vi "Set Laser Power.vi"(6 "Mode":enum16{"Normal", "Ignore", "Reset"}(ring), 7 "Correlation ID":u32, 8 "error in (no error)":errorcluster, 9 "Power":dbl, 10 "laser index":u16, 11 "Application in":refnum<class "Application.lvclass">) -> (0 "error out":errorcluster, 3 "Application out":refnum<class "Application.lvclass">)   [LabVIEW 2023, in "Application.lvlib" / "Application.lvclass"]
uses:
  Application.lvclass
  Application.lvclass/Application.ctl
  Hardware/Device Messages/Save CorrID Msg/Save CorrID Msg.lvclass/Save CorrID Msg.ctl
  <vilib>/ActorFramework/Message Enqueuer/Message Enqueuer.lvclass/Message Enqueuer.ctl
  Hardware/Laser Messages/Set Power Msg/Set Power Msg.lvclass/Set Power Msg.ctl
  <vilib>/ActorFramework/Message Enqueuer/Enqueue.vi
  Hardware/Device Messages/Save CorrID Msg/Save CorrID Msg.lvclass
  Hardware/Laser Messages/Set Power Msg/Set Power Msg.lvclass
  <vilib>/ActorFramework/Message Priority Queue/Priority Enqueue.vi
  Application.lvlib
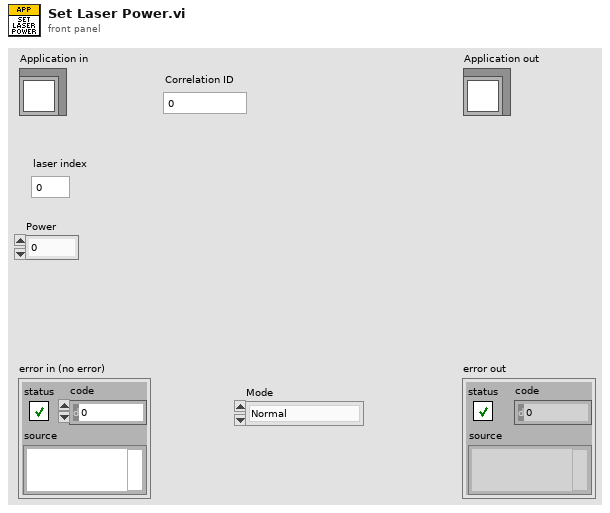
[diagram p1: front panel]
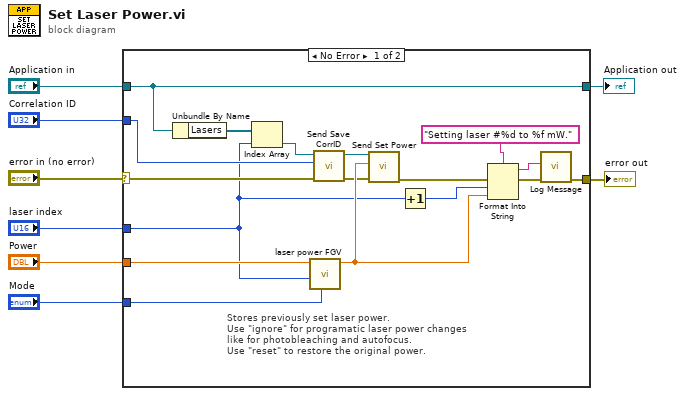
[diagram p0: block diagram]
diagram:
  n1 = case shown="No Error" "error in (no error)" {
    selector: "error in (no error)" -> [w15 w27]
    tunnel: [w22 w27] -> w7
    tunnel: [w12 w26] -> w5
    tunnel: "Application in" -> [w12 w26]
    tunnel: "Power" -> [w25 _]
    tunnel: "laser index" -> [w9 _]
    tunnel: "Mode" -> [w24 _]
    tunnel: "Correlation ID" -> [w13 _]
    frame No Error {
      # "Stores previously set laser power.\nUse \"ignore\" for programatic laser power changes\nlike for photobleaching and autofocus.\nUse \"reset\" to restore the original power."
      n2 = Unbundle By Name(w12) -> ("Lasers"=w23:refnum<class "Message Enqueuer.lvclass">[])
      n3 = Index Array(array=w23, index=w9) -> (element=w16:refnum<class "Message Enqueuer.lvclass">)
      n4 = call "laser power FGV.vi"("Mode"=w24, "laser index"=w9, "Input power"=w25) -> ("Output power"=w18:dbl)  [unwired: 8 in]
      n5 = call "Send Save CorrID.vi"("error in (no error)"=w15, "Correlation ID"=w13, "Message Enqueuer"=w16) -> ("error out"=w14:errorcluster, "Message Enqueuer out"=w17:refnum<class "Message Enqueuer.lvclass">)  [unwired: 7 in]
      n6 = call "Send Set Power.vi"("error in (no error)"=w14, "Power"=w18, "Message Enqueuer"=w17) -> ("error out"=w11:errorcluster)  [unwired: 7 in, 1 out]
      n7 = Increment(x=w9) -> (x+1=w10:u16)
      n8 = Format Into String(format string="Setting laser #%d to %f mW.", error in=w11, w10, w18) -> (resulting string=w20:string, error out=w21:errorcluster)  [unwired: 1 in]
      n9 = call "Log Message.vi"("error constant"=w21, "input"=w20) -> ("error constant 2"=w22:errorcluster)  [unwired: 8 in, 1 out]
    }
    frame Error {
    }
  }
  "error out" <- w7
  "Application out" <- w5
